vi "monostepgf1.vi"(0 "Wait Between Steps(ms)":u8=8, 1 "Steps":i32=1, 2 "Direction":string, 3 "address":i16 format="%.0x") -> ()   [LabVIEW 2010]
uses:
  <vilib>/Platform/portaccess.llb/Out Port32.vi
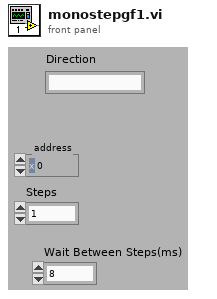
[diagram p1: front panel]
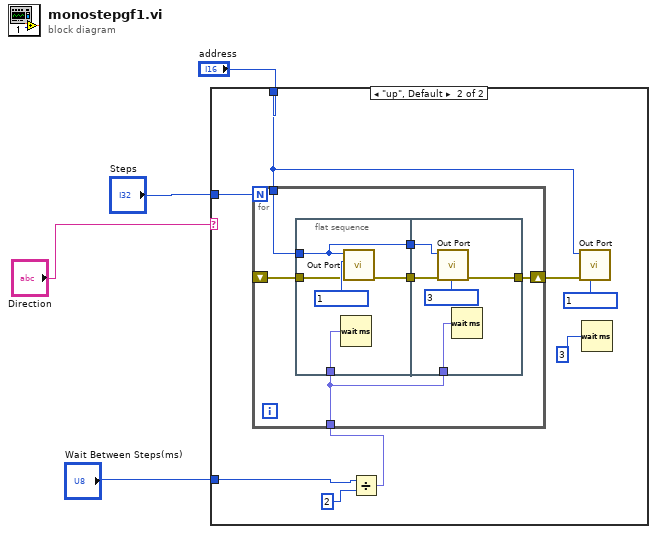
[diagram p0: block diagram]
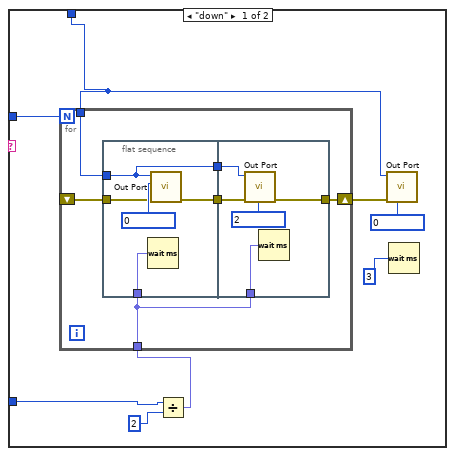
[diagram p2: hidden frame]
diagram:
  n1 = case shown="\"up\", Default" "Direction" {
    tunnel: "Steps" -> [w6 w36]
    tunnel: "address" -> [w5 w33]
    tunnel: "Wait Between Steps(ms)" -> [w7 w30]
    frame "down" {
      n2 = Divide(x=w7, y=u8 2) -> (x/y=w9:fxp<+,8,8>)
      n3 = for {
        N: w6 -> [_]
        shift-right: [w17] -> w11
        shift-left: _ -> [w16]
        tunnel: w5 -> [w15]
        tunnel: w9 -> [w13]
        n4 = flat-sequence {
          tunnel: [w22] -> w18
          tunnel: w16 -> [w21]
          tunnel: w15 -> [w20]
          tunnel: [w20] -> w14
          tunnel: w13 -> [w19]
          tunnel: w18 -> [w28]
          tunnel: [w27] -> w17
          tunnel: w14 -> [w26]
          tunnel: w13 -> [w25]
          frame #0 {
            n5 = Wait (ms)(milliseconds to wait=w19) -> ()  [unwired: 1 out]
            n6 = call-poly <vilib>:"Out Port.vi"("error in (no error)"=w21, "write value"=0, "address"=w20) -> ("error out"=w22:errorcluster)  [unwired: 6 in]
          }
          frame #1 {
            n7 = call-poly <vilib>:"Out Port.vi"("error in (no error)"=w28, "write value"=2, "address"=w26) -> ("error out"=w27:errorcluster)  [unwired: 6 in]
            n8 = Wait (ms)(milliseconds to wait=w25) -> ()  [unwired: 1 out]
          }
        }
      }
      n9 = call-poly <vilib>:"Out Port.vi"("error in (no error)"=w11, "write value"=0, "address"=w5) -> ()  [unwired: 6 in, 1 out]
      n10 = Wait (ms)(milliseconds to wait=u32 3) -> ()  [unwired: 1 out]
    }
    frame "up", Default {
      n11 = Divide(x=w30, y=u8 2) -> (x/y=w31:fxp<+,8,8>)
      n12 = for {
        N: w36 -> [_]
        shift-right: [w41] -> w34
        shift-left: _ -> [w40]
        tunnel: w33 -> [w39]
        tunnel: w31 -> [w37]
        n13 = flat-sequence {
          tunnel: [w46] -> w42
          tunnel: w40 -> [w45]
          tunnel: w39 -> [w44]
          tunnel: [w44] -> w38
          tunnel: w37 -> [w43]
          tunnel: w42 -> [w52]
          tunnel: [w51] -> w41
          tunnel: w38 -> [w50]
          tunnel: w37 -> [w49]
          frame #0 {
            n14 = Wait (ms)(milliseconds to wait=w43) -> ()  [unwired: 1 out]
            n15 = call-poly <vilib>:"Out Port.vi"("error in (no error)"=w45, "write value"=1, "address"=w44) -> ("error out"=w46:errorcluster)  [unwired: 6 in]
          }
          frame #1 {
            n16 = call-poly <vilib>:"Out Port.vi"("error in (no error)"=w52, "write value"=3, "address"=w50) -> ("error out"=w51:errorcluster)  [unwired: 6 in]
            n17 = Wait (ms)(milliseconds to wait=w49) -> ()  [unwired: 1 out]
          }
        }
      }
      n18 = call-poly <vilib>:"Out Port.vi"("error in (no error)"=w34, "write value"=1, "address"=w33) -> ()  [unwired: 6 in, 1 out]
      n19 = Wait (ms)(milliseconds to wait=u32 3) -> ()  [unwired: 1 out]
    }
  }
